vi "Page_Info_Update_Main_Destination_Name.vi"(8 "error in (no error)":errorcluster, 10 "destination name":string, 11 "AB_RESTfulWebService in":refnum<class "AB_RESTfulWebService.lvclass">) -> (0 "error out":errorcluster, 3 "AB_RESTfulWebService out":refnum<class "AB_RESTfulWebService.lvclass">)   [LabVIEW 2020, in "AB_RESTfulWebService.lvclass"]
uses:
  <vilib>/AppBuilder/AB_Classes/RESTful/AB_RESTfulWebService.lvclass
  <vilib>/AppBuilder/AB_Classes/RESTful/AB_RESTfulWebService.lvclass/AB_RESTfulWebService.ctl
  <vilib>/AppBuilder/AB_Classes/WebService/AB_WebService.lvclass
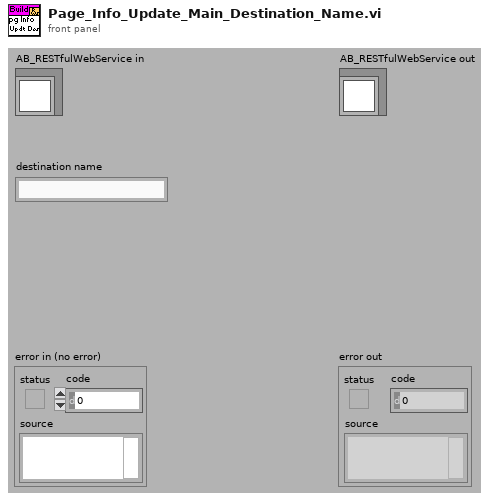
[diagram p1: front panel]
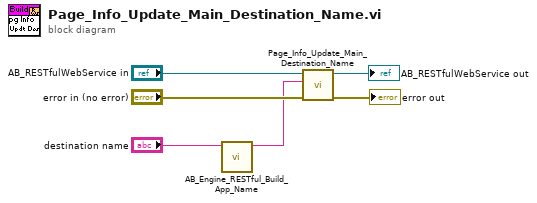
[diagram p0: block diagram]
diagram:
  n1 = call <vilib>:"AB_Engine_RESTful_Build_App_Name.vi"("service name"="destination name") -> ("app name"=w1:string)  [unwired: 10 in]
  n2 = call-parent "Page_Info_Update_Main_Destination_Name.vi"("error in (no error)"="error in (no error)", "destination name"=w1, "AB_Build in"="AB_RESTfulWebService in") -> ("error out"=→"error out":errorcluster, "AB_Build out"=→"AB_RESTfulWebService out":refnum<class "AB_RESTfulWebService.lvclass">)  [unwired: 7 in]
